vi "DIOSerialPort.vi"(11 "DIOSerialPortSettings":T1={"TxPort"="ModbusPort1Tx", "TxDataFIFO"="ModbusPort1TxFIFO", "RxPort"="ModbusPort1Rx", "RxDataFIFO"="ModbusPort1RxFIFO"}) -> ()   [LabVIEW 2018]
uses:
  DIOSerialPortSettings.ctl
  <vilib>/rvi/eio/common/nirviEmuTemplateMethod_errors.vi
  <vilib>/rvi/Emulation/niFpgaProcessEmulError.vi
  <vilib>/eio/EIONode/EIONode.xnode
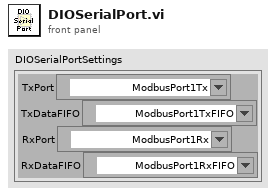
[diagram p1: front panel]
types:
  T1 = typedef "DIOSerialPortSettings.ctl" = cluster{"TxPort":refnum<k21>, "TxDataFIFO":refnum<k21>, "RxPort":refnum<k21>, "RxDataFIFO":refnum<k21>}
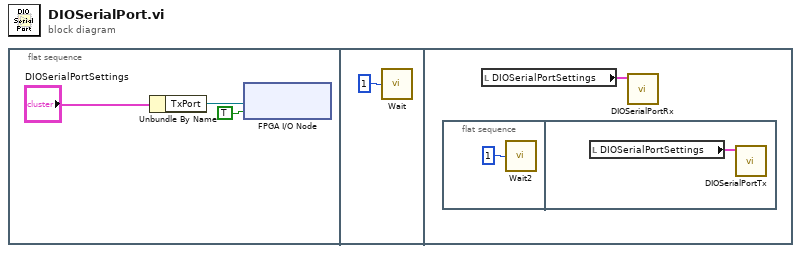
[diagram p0: block diagram]
diagram:
  n1 = flat-sequence {
    frame #0 {
      n2 = Unbundle By Name("DIOSerialPortSettings") -> ("TxPort"=w2:refnum<k21>)
      n3 = xnode "FPGA I/O Node"("I/O Item"=TRUE, "FPGA I/O In"=w2) -> ()  [unwired: 1 out]
    }
    frame #1 {
      n4 = call "Wait"("Count(mSec)"=u8 1 ("Count(Ticks)")) -> ()  [unwired: 1 out]
    }
    frame #2 {
      n5 = flat-sequence {
        frame #0 {
          n6 = call "Wait2"("Count(mSec)"=u8 1 ("Count(Ticks)")) -> ()  [unwired: 1 out]
        }
        frame #1 {
          n7 = local read "DIOSerialPortSettings"() -> (w7:T1)
          n8 = call "DIOSerialPortTx.vi"("DIOSerialPortSettings"=w7) -> ()  [unwired: 11 in]
        }
      }
      n9 = local read "DIOSerialPortSettings"() -> (w5:T1)
      n10 = call "DIOSerialPortRx.vi"("DIOSerialPortSettings"=w5) -> ()  [unwired: 11 in]
    }
  }
